vi "Day 4 (Part One).vi"() -> ()   [LabVIEW 2021]
panel:
  out "sum":i16
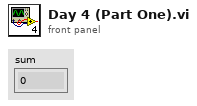
[diagram p1: front panel]
types:
  T1 = cluster{"Range A_Low":i32, "Range A_High":i32, "Range B_Low":i32, "Range B_High":i32}
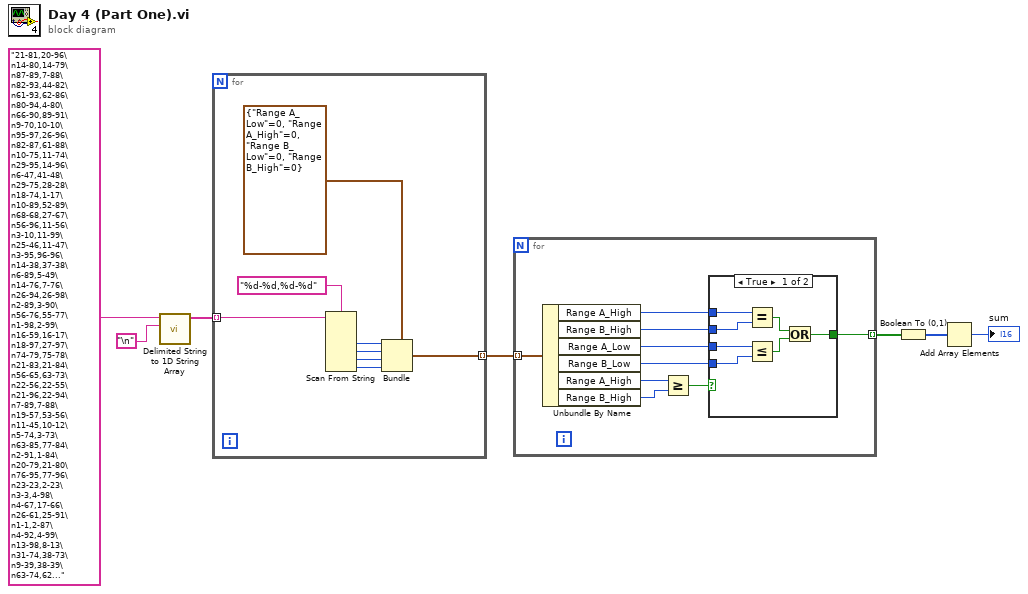
[diagram p0: block diagram]
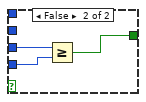
[diagram p2: hidden frame]
diagram:
  n1 = call <vilib>:"Delimited String to 1D String Array.vi"("delimiter"="\n", "delimited string"="21-81,20-96\n14-80,14-79\n87-89,7-88\n82-93,44-82\n61-93,62-86\n80-94,4-80\n66-90,89-91\n9-70,10-10\n95-97,26-96\n82-87,61-88\n10-75,11-74\n29-95,14-96\n6-47,41-48\n29-75,28-28\n18-74,1-17\n10-89,52-89\n68-68,27-67\n56-96,11-56\n3-10,11-99\n25-46,11-47\n3-95,96-96\n14-38,37-38\n6-89,5-49\n14-76,7-76\n26-94,26-98\n2-89,3-90\n56-76,55-77\n1-98,2-99\n16-59,16-17\n18-97,27-97\n74-79,75-78\n21-83,21-84\n56-65,63-73\n22-56,22-55\n21-96,22-94\n7-89,7-88\n19-57,53-56\n11-45,10-12\n5-74,3-73\n63-85,77-84\n2-91,1-84\n20-79,21-80\n76-95,77-96\n23-23,2-23\n3-3,4-98\n4-67,17-66\n26-61,25-91\n1-1,2-87\n4-92,4-99\n13-98,8-13\n31-74,38-73\n9-39,38-39\n63-74,62-74\n65-91,9-64\n1-85,1-86\n14-22,23-23\n19-78,79-79\n24-42,25-41\n10-54,9-9\n6-96,3-4\n39-97,38-38\n48-58,59-77\n13-13,14-22\n97-98,3-98\n10-92,9-9\n69-71,77-90\n1-99,99-99\n24-25,25-82\n8-92,3-8\n20-91,19-98\n34-89,90-90\n56-56,56-95\n16-17,17-80\n13-97,10-99\n10-98,10-88\n13-76,76-77\n8-70,15-69\n15-95,95-95\n21-37,27-36\n53-64,7-52\n15-84,34-84\n60-60,17-60\n5-94,2-3\n1-1,2-90\n68-70,70-97\n62-64,4-63\n6-97,5-98\n77-90,73-77\n21-22,22-23\n91-97,96-97\n11-96,12-28\n42-63,42-62\n31-73,14-81\n72-72,4-71\n10-75,9-76\n7-7,8-89\n51-96,52-97\n23-32,5-33\n2-82,2-83\n1-99,91-98\n6-95,7-94\n16-63,16-17\n65-95,99-99\n3-98,56-97\n82-84,1-83\n89-89,67-88\n37-70,95-97\n33-34,4-33\n4-92,63-92\n3-88,2-88\n14-93,13-13\n34-36,35-70\n10-32,31-75\n8-38,7-38\n43-54,43-62\n6-8,7-14\n5-99,1-98\n29-52,51-52\n12-58,44-84\n18-96,19-35\n19-37,18-20\n2-3,3-3\n1-55,1-56\n94-97,20-75\n44-86,98-98\n20-61,88-92\n28-92,13-78\n49-95,50-50\n18-62,61-63\n47-81,46-82\n12-59,12-60\n77-77,27-77\n6-91,5-64\n87-87,1-86\n6-23,6-22\n13-99,13-98\n69-98,13-96\n3-68,2-95\n28-87,31-88\n26-91,25-94\n6-78,31-77\n12-85,12-69\n25-27,26-26\n60-60,11-60\n18-97,1-96\n3-96,2-95\n1-95,2-93\n17-49,34-68\n3-56,1-4\n2-99,25-97\n4-80,2-5\n6-79,10-87\n16-18,14-21\n42-79,80-80\n20-59,21-58\n98-99,75-99\n55-73,24-74\n10-93,9-11\n65-80,64-79\n39-96,11-39\n31-96,31-76\n2-94,1-3\n7-29,91-96\n20-53,18-20\n47-68,32-48\n4-13,14-28\n49-56,18-57\n55-65,65-73\n27-64,65-83\n40-40,16-40\n48-67,40-48\n24-91,43-92\n16-68,36-69\n2-2,1-50\n5-8,7-47\n40-88,2-40\n40-90,40-40\n11-62,12-68\n16-69,15-80\n19-71,70-94\n9-79,9-80\n17-96,97-97\n23-97,23-99\n25-25,13-25\n33-40,32-39\n58-60,14-59\n3-59,2-2\n34-40,35-35\n35-35,29-34\n16-87,17-88\n16-26,42-84\n26-68,25-26\n36-82,37-90\n20-20,20-20\n5-26,10-25\n22-52,6-23\n18-97,97-97\n5-51,6-6\n37-53,24-87\n13-18,18-24\n67-95,80-86\n2-14,13-42\n40-70,9-63\n14-54,14-53\n3-7,3-6\n11-42,16-93\n1-97,21-87\n67-74,68-72\n20-98,19-98\n18-33,29-33\n48-94,95-95\n72-92,46-77\n16-92,92-94\n44-46,45-75\n34-94,94-94\n31-80,80-80\n10-31,32-99\n6-41,15-42\n20-20,19-77\n12-95,7-9\n35-36,2-38\n10-21,9-9\n10-58,11-11\n16-37,17-37\n69-73,29-69\n82-86,41-85\n71-93,72-85\n44-82,43-98\n40-96,23-96\n12-97,12-96\n86-88,10-97\n54-81,80-81\n9-19,9-71\n32-83,83-84\n32-89,31-98\n60-84,60-83\n92-93,7-93\n17-99,17-97\n19-49,19-48\n24-48,45-47\n6-40,7-39\n6-89,6-67\n83-88,82-88\n3-98,3-99\n4-4,3-92\n4-41,40-95\n53-87,88-88\n63-65,61-64\n7-73,7-7\n25-25,26-47\n31-98,50-99\n32-96,27-33\n55-57,34-56\n1-9,9-97\n20-72,7-20\n6-6,5-59\n28-44,43-45\n97-97,14-96\n69-69,47-68\n39-40,39-54\n19-49,47-67\n54-96,29-53\n79-96,64-80\n52-70,53-63\n17-90,17-57\n12-28,27-36\n23-76,94-98\n46-53,47-47\n31-57,30-89\n14-57,37-45\n2-99,1-99\n92-93,92-93\n5-92,5-83\n20-97,74-98\n14-27,27-80\n2-74,2-98\n24-35,34-45\n47-48,13-48\n29-71,26-71\n39-39,40-69\n2-50,49-51\n29-47,26-32\n12-48,11-11\n1-64,2-63\n16-63,6-16\n12-89,89-89\n37-63,38-62\n8-54,6-8\n1-98,4-95\n28-76,69-83\n5-79,6-80\n6-6,7-96\n16-80,16-16\n48-96,49-91\n17-90,18-90\n22-27,27-27\n72-90,67-91\n7-7,8-89\n90-93,36-90\n70-72,53-73\n14-91,15-92\n31-99,98-99\n31-68,30-95\n43-74,42-98\n23-32,28-34\n19-19,18-54\n15-15,6-15\n24-81,25-25\n9-85,8-85\n3-56,55-77\n16-96,17-18\n10-95,96-96\n4-5,8-15\n11-81,12-80\n43-43,42-48\n12-28,27-85\n33-33,28-33\n2-2,3-97\n85-85,57-84\n12-94,95-98\n26-28,27-67\n35-51,34-51\n12-36,36-36\n31-35,32-44\n1-2,3-89\n13-72,12-75\n2-59,2-58\n10-85,84-86\n38-95,45-59\n8-93,93-93\n97-98,9-98\n17-92,5-9\n34-87,89-92\n24-43,44-63\n3-99,1-3\n26-64,27-64\n41-41,40-85\n33-82,4-34\n10-98,99-99\n1-83,2-84\n55-91,55-86\n2-13,7-32\n3-3,2-76\n73-92,9-73\n3-6,5-7\n10-44,14-43\n10-89,9-11\n74-76,17-75\n8-11,1-11\n50-58,97-97\n66-86,65-65\n5-68,69-69\n5-5,6-59\n2-14,8-93\n36-91,97-97\n55-74,74-84\n41-84,40-91\n16-75,6-76\n17-85,88-94\n27-33,32-34\n63-64,4-64\n27-93,27-92\n31-78,30-77\n16-37,43-87\n14-94,14-71\n24-98,23-24\n19-94,95-95\n98-98,53-76\n9-86,2-10\n53-53,34-52\n34-42,34-36\n26-91,24-90\n90-96,90-95\n11-88,12-50\n45-81,31-44\n6-38,5-39\n35-51,34-50\n54-68,68-95\n16-70,6-10\n29-81,82-82\n20-93,34-94\n50-97,84-97\n92-98,53-68\n44-52,43-52\n15-96,27-97\n47-47,46-63\n54-90,53-53\n20-55,20-56\n5-74,30-75\n2-64,7-65\n7-83,8-82\n45-49,14-59\n1-74,12-75\n10-98,11-98\n26-99,25-89\n28-99,29-29\n23-65,22-91\n7-7,6-10\n22-46,42-50\n25-67,67-79\n42-81,32-82\n35-96,34-35\n1-99,99-99\n7-40,8-41\n43-62,44-93\n82-82,6-81\n74-99,7-73\n5-87,6-6\n44-80,4-81\n24-30,56-71\n33-60,32-60\n11-78,1-79\n6-41,6-6\n51-55,52-54\n49-51,42-50\n47-60,19-47\n46-81,47-96\n16-75,16-76\n35-43,43-96\n90-97,17-89\n92-94,31-91\n37-59,21-37\n2-94,6-95\n11-66,11-65\n4-65,2-62\n30-72,71-72\n16-61,61-61\n6-89,26-88\n28-94,94-94\n20-58,20-59\n18-92,94-98\n88-88,89-98\n23-70,23-71\n20-81,20-80\n57-88,14-95\n1-99,2-98\n52-98,21-52\n88-88,5-87\n94-97,87-87\n42-52,43-49\n14-75,15-76\n2-84,37-84\n52-57,49-62\n2-69,3-70\n9-13,13-85\n56-98,57-93\n42-92,29-54\n68-96,67-95\n20-64,19-19\n86-94,65-87\n27-45,46-46\n11-11,11-49\n8-95,16-95\n61-69,62-78\n32-97,32-98\n55-91,28-91\n11-98,12-97\n14-17,19-93\n10-81,54-80\n1-92,17-80\n27-90,28-39\n89-89,4-88\n29-30,21-30\n2-93,94-94\n23-50,24-34\n5-87,18-87\n32-41,33-36\n13-30,13-44\n39-44,38-45\n9-22,8-62\n78-87,32-78\n63-91,63-70\n5-51,45-53\n66-67,24-67\n20-20,20-72\n59-60,6-60\n7-93,8-76\n59-87,32-58\n52-94,53-53\n15-36,36-53\n23-82,6-14\n15-67,5-14\n30-60,30-30\n5-55,32-56\n48-72,6-49\n1-88,20-88\n8-97,9-98\n18-46,17-27\n69-80,81-81\n19-93,21-38\n17-59,58-60\n47-55,40-48\n23-91,91-96\n2-2,1-99\n14-89,89-89\n72-74,28-71\n99-99,2-98\n10-98,7-10\n8-99,9-98\n5-13,12-80\n92-99,1-93\n49-62,50-50\n11-50,11-49\n12-84,5-85\n11-81,9-81\n10-38,10-39\n18-71,14-94\n30-99,98-99\n5-95,3-4\n45-93,28-94\n38-63,39-64\n9-81,6-82\n37-90,58-89\n58-88,60-88\n73-95,33-54\n10-96,11-18\n5-27,4-26\n19-67,20-66\n10-29,9-37\n34-39,32-39\n3-10,10-71\n4-69,6-70\n47-47,48-58\n5-76,96-99\n3-98,4-97\n95-95,4-94\n52-53,47-53\n44-63,11-44\n69-86,60-85\n16-86,15-98\n5-99,6-99\n10-97,97-99\n89-89,4-88\n9-51,52-81\n54-86,54-55\n1-41,2-40\n66-96,16-65\n51-76,76-76\n89-89,89-89\n29-77,30-78\n28-93,27-92\n36-78,90-99\n83-83,84-96\n21-89,89-91\n16-70,8-16\n3-13,5-13\n51-92,11-92\n2-89,1-1\n5-96,2-96\n7-98,99-99\n8-29,1-30\n17-97,17-98\n72-78,53-71\n21-21,22-46\n2-93,7-93\n21-91,21-90\n69-73,30-74\n1-41,4-40\n1-97,1-98\n26-74,25-27\n4-27,26-99\n39-42,38-58\n18-74,6-11\n78-79,65-79\n27-44,45-92\n3-91,1-91\n13-96,14-92\n71-81,78-82\n4-85,27-84\n92-93,11-93\n46-59,46-58\n4-96,1-96\n5-84,6-54\n41-52,42-49\n35-92,66-93\n13-96,13-94\n4-90,1-30\n16-18,17-85\n90-92,46-90\n46-48,47-68\n60-93,42-92\n23-64,64-64\n5-35,24-36\n22-90,21-99\n93-93,90-94\n7-70,64-94\n4-4,5-96\n11-70,5-78\n9-30,7-8\n4-99,45-64\n7-49,7-50\n96-99,64-96\n34-36,35-84\n90-92,21-91\n3-4,5-89\n13-13,12-77\n17-54,20-55\n46-76,76-88\n6-91,90-91\n20-38,5-19\n43-80,22-79\n4-98,97-97\n65-80,71-79\n46-92,13-92\n9-79,9-19\n2-98,2-99\n18-20,21-52\n29-55,54-69\n17-17,16-16\n77-88,24-84\n24-28,22-27\n9-84,84-84\n13-99,13-98\n34-70,69-71\n71-98,98-98\n69-80,69-88\n8-18,18-18\n23-78,79-79\n27-62,28-28\n63-77,41-66\n6-96,7-95\n15-71,23-70\n24-64,20-64\n56-83,13-56\n38-66,37-96\n2-42,1-2\n34-74,64-73\n45-76,45-50\n3-44,1-2\n68-94,68-68\n4-68,69-69\n20-96,96-99\n3-98,1-99\n13-22,23-44\n21-34,26-35\n3-98,4-97\n1-3,4-58\n95-95,74-95\n1-93,1-92\n54-55,22-55\n8-20,7-37\n23-47,16-81\n12-78,13-77\n49-60,50-55\n43-98,64-97\n9-99,9-64\n80-85,53-82\n64-90,13-64\n45-88,33-59\n45-81,46-46\n18-72,18-77\n43-43,44-45\n46-76,77-77\n6-14,13-97\n29-89,7-90\n53-95,7-54\n71-71,71-92\n67-83,84-88\n1-95,96-97\n16-96,8-15\n27-77,77-92\n6-58,5-59\n50-85,51-57\n83-84,36-83\n66-80,53-75\n80-80,60-79\n4-91,4-28\n56-70,30-69\n34-52,36-52\n20-87,86-88\n25-44,40-44\n58-87,8-59\n31-92,31-93\n4-54,4-71\n8-57,18-57\n11-46,47-47\n36-49,30-50\n3-86,1-15\n2-78,3-77\n82-82,4-82\n22-98,2-21\n55-75,42-75\n30-82,46-83\n63-93,64-94\n50-50,19-50\n80-92,79-79\n8-16,7-60\n47-87,14-46\n14-24,24-70\n54-87,55-55\n7-48,6-6\n47-48,40-48\n12-63,63-63\n17-18,18-32\n32-90,44-85\n14-69,6-92\n29-82,18-29\n1-79,18-78\n11-81,5-10\n5-8,9-79\n4-98,5-5\n36-96,94-97\n12-64,26-63\n28-84,27-28\n11-89,11-88\n31-55,52-54\n3-25,3-55\n76-85,75-91\n23-82,49-93\n24-38,17-38\n56-94,67-93\n10-51,23-52\n24-77,12-76\n54-60,56-59\n25-28,28-28\n49-75,57-74\n10-69,5-7\n45-54,24-49\n11-34,26-33\n29-95,29-99\n9-66,9-87\n3-61,54-62\n46-96,43-68\n9-58,10-78\n22-96,95-96\n2-35,3-34\n3-94,4-95\n78-84,79-85\n93-94,15-94\n23-23,24-89\n13-94,12-94\n4-81,2-80\n6-99,17-99\n26-63,16-63\n8-10,7-13\n23-85,85-85\n70-98,69-99\n26-44,41-43\n17-97,16-97\n62-98,99-99\n46-88,78-87\n18-71,4-18\n96-96,75-96\n37-87,5-86\n14-31,26-30\n23-52,23-75\n16-94,17-17\n50-50,50-50\n9-12,12-98\n98-99,24-99\n7-14,13-55\n14-76,9-76\n11-81,8-82\n89-89,3-89\n13-90,14-84\n7-86,86-86\n2-8,7-50\n11-98,11-99\n13-96,96-96\n5-8,8-50\n10-54,11-53\n6-75,7-72\n50-51,15-51\n7-37,9-37\n34-35,18-61\n11-76,10-84\n4-62,1-3\n1-87,20-84\n7-83,8-87\n5-14,7-51\n56-58,10-57\n2-2,3-92\n56-68,37-85\n57-57,52-56\n40-79,78-79\n73-74,4-74\n8-98,99-99\n76-76,70-77\n79-94,66-78\n10-68,11-65\n10-24,23-42\n82-83,46-83\n54-92,55-91\n7-17,18-60\n50-80,58-81\n75-77,76-76\n1-99,2-55\n91-91,12-91\n1-90,89-91\n22-23,21-42\n80-80,31-80\n6-6,5-20\n34-47,34-78\n2-95,2-99\n30-65,62-65\n10-69,68-70\n8-29,23-43\n37-47,36-49\n62-63,48-63\n21-97,3-97\n25-75,22-25\n92-92,14-92\n94-96,12-94\n1-80,1-81\n27-32,31-33\n26-59,25-88\n86-92,38-86\n34-42,35-41\n58-91,57-95\n62-62,5-62\n3-46,47-73\n13-97,10-37\n9-39,3-10\n55-89,55-81\n41-88,40-40\n22-87,5-88\n78-94,30-78\n86-86,85-86\n5-62,11-90\n46-56,47-55\n4-12,11-92\n99-99,14-98\n9-30,8-80\n43-43,42-45\n53-56,40-56\n3-97,2-97\n13-32,12-95\n10-91,11-92\n86-98,59-87\n6-81,82-82\n24-84,85-87\n39-86,40-40\n31-54,53-75\n7-98,4-87\n70-75,72-74\n29-87,28-98\n26-91,25-25\n12-57,13-56\n19-87,86-88\n9-15,10-16\n12-50,45-65\n53-64,64-64\n90-91,4-91\n2-85,22-85\n13-13,14-87\n30-51,28-29\n17-67,16-93\n14-70,23-68\n65-72,60-71\n5-77,1-78\n10-15,4-11\n2-63,62-64\n4-91,4-80\n24-60,8-59\n1-99,75-98\n11-86,85-86\n16-18,17-91\n50-76,76-78\n54-58,57-59\n13-64,64-70\n15-21,14-25\n23-25,9-24\n40-67,41-68\n16-18,17-95\n59-83,82-83\n45-99,17-42\n8-30,31-75\n1-98,97-98\n2-78,2-77\n19-57,18-19\n25-73,25-59\n21-98,21-95\n14-70,15-54\n81-83,67-82\n1-99,93-98\n8-35,35-83\n2-83,2-84\n7-96,6-99\n11-63,11-64\n46-80,17-94\n4-61,3-62\n54-97,55-97\n73-73,21-73\n6-66,65-67\n56-89,61-88\n42-53,41-70\n5-46,5-45\n46-92,20-91\n93-96,15-93\n57-64,52-65\n28-28,27-87\n8-47,2-7\n31-31,32-33\n1-99,2-97\n12-84,83-84\n3-14,15-90\n8-8,8-64\n35-85,14-36\n83-99,58-98\n4-93,3-99\n26-77,18-27\n1-83,21-27\n95-95,16-94\n5-66,6-27\n66-84,21-78\n40-85,43-86\n19-75,12-19\n11-96,1-10\n40-53,20-40\n29-57,45-79\n36-75,35-35\n10-10,5-10\n62-78,70-77\n2-95,11-94\n37-37,36-89\n5-15,1-19\n73-96,82-96\n27-27,26-82\n91-93,27-92\n62-74,21-62\n29-35,36-85\n29-33,28-96\n60-92,26-61\n1-86,1-86\n6-8,9-44\n3-68,25-67\n2-12,13-32\n3-71,72-72\n47-93,14-47\n34-88,60-95\n6-28,28-93\n37-62,33-38\n8-93,8-92\n9-15,15-77\n38-44,39-39\n5-88,4-4\n17-94,16-18\n84-84,7-83\n1-4,4-29\n27-80,12-79\n3-78,78-78\n76-79,75-77\n2-94,96-98\n30-57,20-30\n6-26,27-97\n22-76,21-21\n8-42,9-23\n31-39,38-40\n34-35,5-35\n77-80,76-80\n12-92,11-94\n47-51,12-47\n90-93,37-90\n96-97,12-93\n10-93,1-9\n4-10,3-19\n59-82,60-81\n11-39,10-10\n58-72,59-69\n71-71,70-70\n69-71,71-72\n94-96,4-95\n14-83,5-84\n1-59,12-58\n20-99,98-99\n43-43,42-88\n99-99,51-99\n12-21,11-20\n47-48,22-48\n9-37,9-38\n24-60,24-74\n94-94,2-94\n57-57,58-90\n67-89,66-93\n1-54,11-88\n4-11,12-12\n60-99,60-98\n45-59,53-59\n4-4,3-84\n9-80,8-81\n13-45,14-74\n84-86,73-85\n45-79,44-78\n9-16,9-18\n84-93,93-93\n70-80,71-81\n66-91,39-92\n26-26,27-96\n16-35,35-35\n62-62,62-97\n18-93,19-92\n94-96,64-94\n5-98,2-5\n96-96,95-98\n7-65,2-7\n3-87,4-4\n26-79,56-80\n7-78,7-63\n7-96,3-8\n28-96,28-28") -> ("string array"=w5:string[])  [unwired: 9 in]
  n2 = for {
    tunnel: w5 -> [w15] mode=indexing
    tunnel: [w8] -> w4 mode=indexing
    n3 = Scan From String(format string="%d-%d,%d-%d", input string=w15) -> (output 1=w12:i32, output 2=w11:i32, output 3=w10:i32, output 4=w9:i32)  [unwired: 6 in, 3 out]
    n4 = Bundle(cluster=T1 {"Range A_Low"=0, "Range A_High"=0, "Range B_Low"=0, "Range B_High"=0}, "Range A_Low"=w12, "Range A_High"=w11, "Range B_Low"=w10, "Range B_High"=w9) -> (w8:T1)
  }
  n5 = for {
    tunnel: w4 -> [w19] mode=indexing
    tunnel: [w18] -> w3 mode=indexing
    n6 = Unbundle By Name(w19) -> ("Range A_High"=w17:i32, "Range B_High"=w16:i32, "Range A_Low"=w21:i32, "Range B_Low"=w20:i32, "Range A_High"=w24:i32, "Range B_High"=w23:i32)
    n7 = Greater Or Equal?(x=w24, y=w23) -> (x >= y?=w22:bool)
    n8 = case shown="True" w22 {
      tunnel: w21 -> [w31 w34]
      tunnel: w20 -> [w30 w33]
      tunnel: [w25 w32] -> w18
      tunnel: w17 -> [w29 _]
      tunnel: w16 -> [w28 _]
      frame True {
        n9 = Equal?(x=w29, y=w28) -> (x = y?=w27:bool)
        n10 = Less Or Equal?(x=w31, y=w30) -> (x <= y?=w26:bool)
        n11 = Or(x=w27, y=w26) -> (x .or. y?=w25:bool)
      }
      frame False {
        n12 = Greater Or Equal?(x=w34, y=w33) -> (x >= y?=w32:bool)
      }
    }
  }
  n13 = Boolean To (0,1)(Boolean=w3) -> (0, 1=w2:i16[])
  n14 = Add Array Elements(numeric array=w2) -> (sum=→"sum":i16)
